vi "RS_SMBV100A_arrayStringToDOUBLE.vi"(0 "string":string=" 160440.763,3748.4891,14458.0082,10.4,110.4,line\n 160441.763,3748.4890,14458.0150,10.4,110.4,line\n 160442.763,3748.4889,14458.0227,10.5,110.5,line\n 160443.763,3748.4888,14458.0314,10.5,110.5,line\n 160444.763,3748.4887,14458.0411,10.5,110.5,line\n 160445.763,3748.4887,14458.0518,10.4,110.4,line\n 160446.763,3748.4887,14458.0635,10.5,110.5,line\n 160447.763,3748.4886,14458.0761,10.5,110.5,line\n 160448.762,3748.4886,14458.0897,10.5,110.5,line\n 160449.763,3748.4886,14458.1044,10.5,110.5,line\n 160450.763,3748.4887,14458.1200,10.5,110.5,line\n 160451.763,3748.4887,14458.1366,10.6,110.6,line\n 160452.763,3748.4887,14458.1541,10.6,110.6,line\n 160453.763,3748.4887,14458.1726,10.6,110.6,line\n 160454.763,3748.4888,14458.1915,10.6,110.6,line\n 160455.763,3748.4888,14458.2103,10.6,110.6,line\n 160456.763,3748.4889,14458.2292,10.6,110.6,line\n 160457.763,3748.4889,14458.2482,10.6,110.6,line\n 160458.763,3748.4890,14458.2671,10.6,110.6,line\n 160459.763,3748.4890,14458.2861,10.6,110.6,line\n 160500.763,3748.4891,14458.3050,10.7,110.7,line\n 160501.763,3748.4891,14458.3240,10.7,110.7,line\n 160502.763,3748.4892,14458.3430,10.7,110.7,line\n 160503.763,3748.4892,14458.3620,10.7,110.7,line\n 160504.762,3748.4893,14458.3810,10.7,110.7,line\n 160505.763,3748.4893,14458.4001,10.7,110.7,line\n 160506.763,3748.4894,14458.4191,10.7,110.7,line\n 160507.763,3748.4894,14458.4381,10.7,110.7,line\n 160508.763,3748.4895,14458.4572,10.7,110.7,line", 1 "error in":errorcluster {"code" format="%.0x"}) -> (2 "Dynam waypoints":T1 {"Time" format="%<%.3X>T"; "Speed" format="%#.10g"; "Heigth" format="%#.10g"; "Longitude" format="%#.10g"; "Latitude" format="%#.10g"}, 4 "error out":errorcluster {"code" format="%.0x"})   [LabVIEW 2018]
uses:
  RS_SMBV100A_DynamWaypoints.ctl
  RS_SMBV100A_DynamWaypoint.ctl
panel:
  out "Scenarious name":string[](array[string])
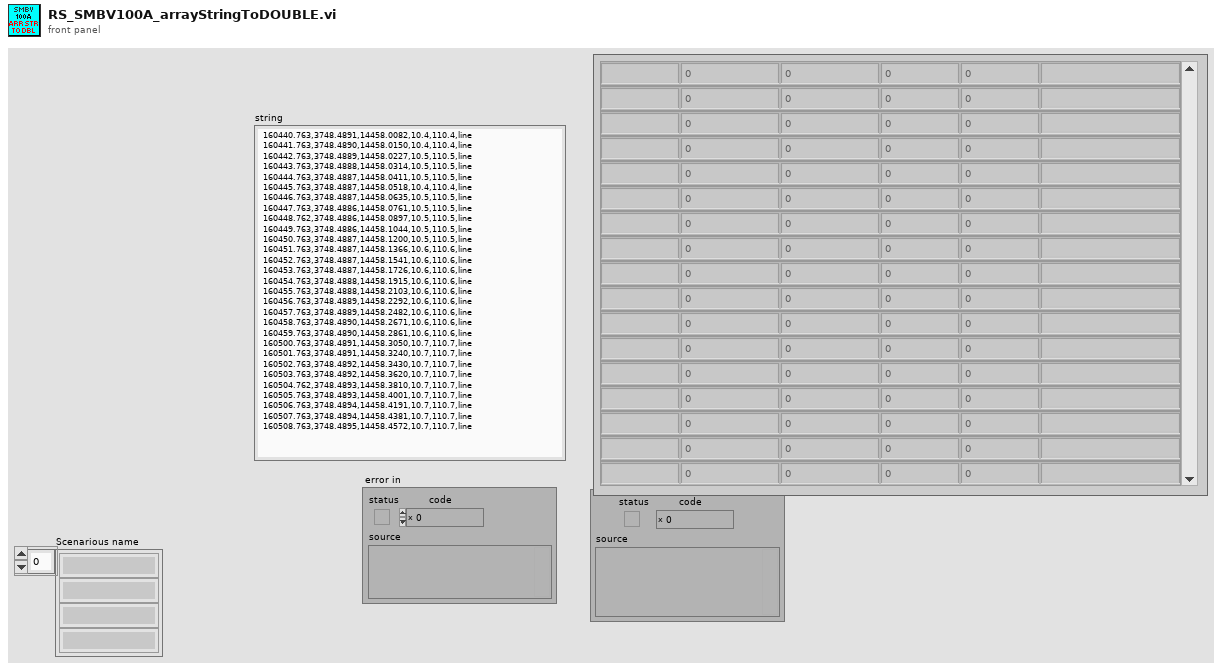
[diagram p1: front panel]
types:
  T1 = typedef "RS_SMBV100A_DynamWaypoints.ctl" = T2[]
  T2 = typedef "RS_SMBV100A_DynamWaypoint.ctl" = cluster{"Time":timestamp, "Latitude":ext, "Longitude":ext, "Heigth":dbl, "Speed":dbl, "Scenario":string}
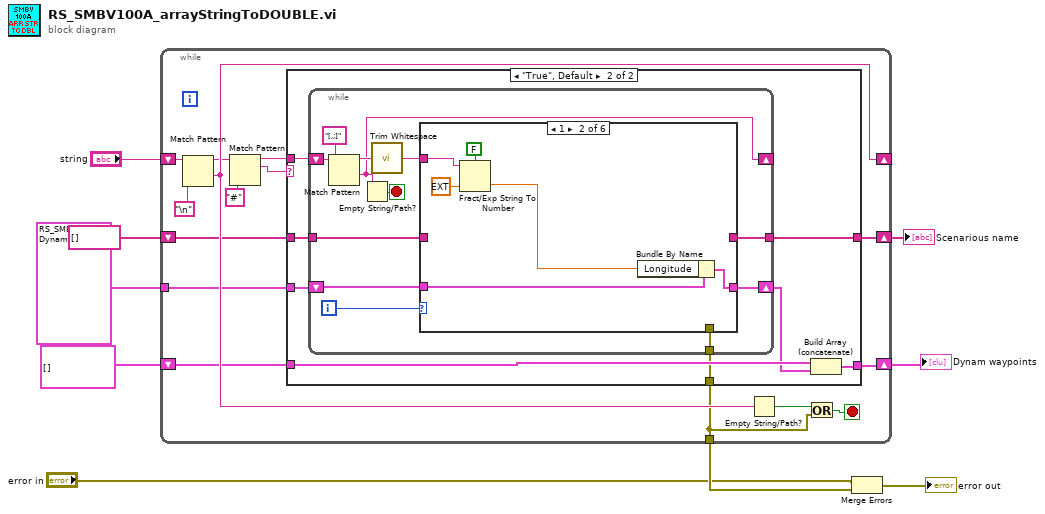
[diagram p0: block diagram]
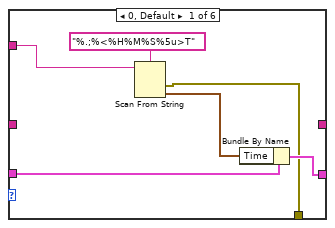
[diagram p3: hidden frame]
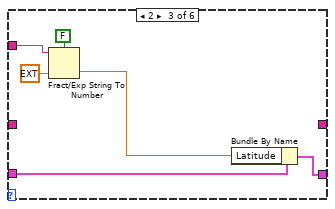
[diagram p4: hidden frame]
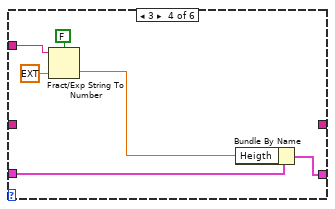
[diagram p5: hidden frame]
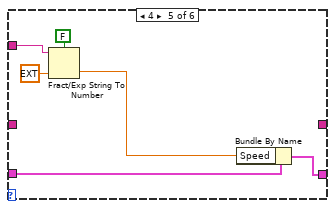
[diagram p6: hidden frame]
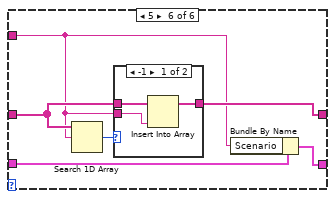
[diagram p7: hidden frame]
diagram:
  n1 = while {
    shift-right: [w22] -> _
    shift-left: "string" -> [w23]
    shift-right: [w15] -> w7
    shift-left: T1 [] ("Dynam waypoints") -> [w16]
    tunnel: T2 {"Time"=timestamp(0 s since 1904-01-01), "Latitude"=0.0, "Longitude"=0.0, "Heigth"=0.0, "Speed"=0.0, "Scenario"=""} ("Cluster") -> [w21]
    tunnel: [w12] -> w6
    shift-right: [w10] -> w4
    shift-left: string[] [] -> [w11]
    stop <- w13 stop-if-true
    n2 = Match Pattern(string=w23, regular expression="\n") -> (before substring=w19:string, after substring=w22:string)  [unwired: 1 in, 2 out]
    n3 = Match Pattern(string=w19, regular expression="#") -> (before substring=w18:string, match substring=w17:string)  [unwired: 1 in, 2 out]
    n4 = case shown="\"True\", Default" w17 {
      tunnel: w21 -> [_ w34]
      tunnel: w18 -> [_ w33]
      tunnel: w16 -> [w26 w32]
      tunnel: [w26 w31] -> w15
      tunnel: [_ w29] -> w12
      tunnel: w11 -> [w25 w28]
      tunnel: [w25 w27] -> w10
      frame "#" {
      }
      frame "True", Default {
        n5 = while {
          shift-right: [w40] -> _
          shift-left: w33 -> [w45]
          shift-right: [w43] -> w30
          shift-left: w34 -> [w44]
          tunnel: [w37] -> w29
          tunnel: w28 -> [w35]
          tunnel: [w36] -> w27
          i -> [w38]
          stop <- w41 stop-if-true
          n6 = Match Pattern(string=w45, regular expression="[,;]") -> (before substring=w42:string, after substring=w40:string)  [unwired: 1 in, 2 out]
          n7 = Empty String/Path?(string/path=w40) -> (empty?=w41:bool)
          n8 = call <vilib>:"Trim Whitespace.vi"("string"=w42) -> ("trimmed string"=w39:string)  [unwired: 1 in]
          n9 = case shown="1" w38 {
            tunnel: w44 -> [w50 w58 w64 w70 w76 w82]
            tunnel: [w49 w57 w63 w69 w75 w81] -> w43
            tunnel: w39 -> [w51 w54 w60 w66 w72 w77]
            tunnel: [w48 _ _ _ _ _] -> w37
            tunnel: [_ _ _ _ _ w79] -> w36
            tunnel: w35 -> [_ _ _ _ _ w78]
            frame 0, Default {
              n10 = Scan From String(format string="%.;%<%H%M%S%5u>T", input string=w51) -> (error out=w48:errorcluster, output 1=w47:timestamp)  [unwired: 3 in, 2 out]
              n11 = Bundle By Name(cluster=w50, "Time"=w47) -> (w49:T2)
            }
            frame 1 {
              n12 = Fract/Exp String To Number(use system decimal point (T)=FALSE, string=w54, default (0 dbl)=ext 0.0 ("default (0 DBL)")) -> (number=w53:ext)  [unwired: 1 in, 1 out]
              n13 = Bundle By Name(cluster=w58, "Longitude"=w53) -> (w57:T2)
            }
            frame 2 {
              n14 = Fract/Exp String To Number(use system decimal point (T)=FALSE, string=w60, default (0 dbl)=ext 0.0 ("default (0 DBL)")) -> (number=w59:ext)  [unwired: 1 in, 1 out]
              n15 = Bundle By Name(cluster=w64, "Latitude"=w59) -> (w63:T2)
            }
            frame 3 {
              n16 = Fract/Exp String To Number(use system decimal point (T)=FALSE, string=w66, default (0 dbl)=ext 0.0 ("default (0 DBL)")) -> (number=w65:ext)  [unwired: 1 in, 1 out]
              n17 = Bundle By Name(cluster=w70, "Heigth"=w65) -> (w69:T2)
            }
            frame 4 {
              n18 = Fract/Exp String To Number(use system decimal point (T)=FALSE, string=w72, default (0 dbl)=ext 0.0 ("default (0 DBL)")) -> (number=w71:ext)  [unwired: 1 in, 1 out]
              n19 = Bundle By Name(cluster=w76, "Speed"=w71) -> (w75:T2)
            }
            frame 5 {
              n20 = Search 1D Array(1D array=w78, element=w77) -> (index of element=w80:i32)  [unwired: 1 in]
              n21 = case shown="-1" w80 {
                tunnel: [w84 w86] -> w79
                tunnel: w78 -> [w85 w86]
                tunnel: w77 -> [w83 _]
                frame -1 {
                  n22 = Insert Into Array(array=w85, new element=w83) -> (w84:string[])  [unwired: 1 in]
                }
                frame 1, Default {
                }
              }
              n23 = Bundle By Name(cluster=w82, "Scenario"=w77) -> (w81:T2)
            }
          }
        }
        n24 = Build Array (concatenate)(w32, w30) -> (w31:T1)
      }
    }
    n25 = Empty String/Path?(string/path=w22) -> (empty?=w14:bool)
    n26 = Or(x=w14, y=w12) -> (x .or. y?=w13:bool)
  }
  "Dynam waypoints" <- w7
  "Scenarious name" <- w4
  n27 = Merge Errors("error in", w6) -> (→"error out":errorcluster)
